vi "Request Logger.vi"(8 "error in (no error)":errorcluster, 11 "Producer in":refnum<class "Log Producer.lvclass">) -> (0 "error out":errorcluster, 3 "Producer out":refnum<class "Log Producer.lvclass">)   [LabVIEW 2024, in "AIM ARINC 429 Engine.lvlib" / "Implementation.lvlib" / "Word Logging.lvlib"]
uses:
  Word Logging.lvlib
  Log Producer/Log Producer.lvclass
  C:/Program Files/National Instruments/LabVIEW 2024/vi.lib/NI/VeriStand Custom Device Messaging/Producer/Abstract Producer/Abstract Producer.lvclass
  <vilib>/NI/VeriStand Custom Device Messaging/Consumer/Abstract Consumer/Abstract Consumer.lvclass
  <vilib>/NI/VeriStand Custom Device Messaging/Message Queue/Message Queue/Message Queue.lvclass
  C:/Program Files/National Instruments/LabVIEW 2024/vi.lib/NI/VeriStand Custom Device Messaging/Message Queue/Abstract Message Queue/Abstract Message Queue.lvclass
  <vilib>/NI/VeriStand Custom Device Messaging/Parameters/Abstract Init Parameters/Abstract Init Parameters.lvclass
  <vilib>/NI/VeriStand Custom Device Messaging/Producer/Abstract Producer/Abstract Producer.lvclass
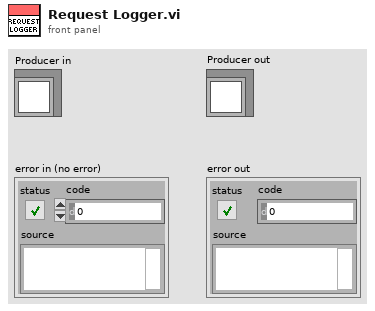
[diagram p1: front panel]
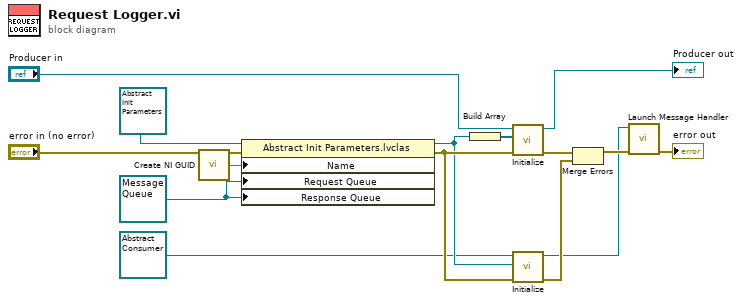
[diagram p0: block diagram]
diagram:
  w13 = refnum<class "Message Queue.lvclass"> refnum ("Messaging.lvlib:Message Queue.lvclass")
  n1 = call <vilib>:"Create NI GUID.vi"() -> ("NI GUID"=w12:string)
  n2 = property class="Abstract Init Parameters.lvclas"(reference=refnum<class "Abstract Init Parameters.lvclass"> refnum ("Messaging.lvlib:Abstract Init Parameters.lvclass"), error in="error in (no error)", "Name"=w12, "Request Queue"=w13, "Response Queue"=w13) -> (reference out=w7:refnum<class "Abstract Init Parameters.lvclass">, error out=w15:errorcluster)
  n3 = Build Array(w7) -> (w8:refnum<class "Abstract Init Parameters.lvclass">[])
  n4 = call <vilib>:"Initialize.vi"("error in (no error)"=w15, "Parameters in"=w8, "Abstract Producer in"="Producer in") -> ("error out"=w11:errorcluster, "Abstract Producer out"=→"Producer out":refnum<class "Log Producer.lvclass">)  [unwired: 7 in]
  n5 = call <vilib>:"Initialize.vi"("error in (no error)"=w15, "Parameters in"=w7, "Abstract Consumer in"=refnum<class "Abstract Consumer.lvclass"> refnum ("Messaging.lvlib:Abstract Consumer.lvclass")) -> ("error out"=w10:errorcluster, "Abstract Consumer out"=w2:refnum<class "Abstract Consumer.lvclass">)  [unwired: 7 in]
  n6 = Merge Errors(w11, w10) -> (w4:errorcluster)
  n7 = call "Launch Message Handler.vi"("error in (no error)"=w4, "Consumer"=w2) -> ("error out"=→"error out":errorcluster)  [unwired: 9 in]
